vi "get_dequeue_buffer_element.vi"(8 "error in (no error)":errorcluster, 10 "continuous samples?":i32, 11 "SignalWriterMH110203USBStepperMotor in":refnum<class "SignalWriterMH110203USBStepperMotor.lvclass">) -> (0 "error out":errorcluster, 1 "finished?":bool, 2 "dequeued element":dbl, 3 "SignalWriterMH110203USBStepperMotor out":refnum<class "SignalWriterMH110203USBStepperMotor.lvclass">)   [LabVIEW 2010, in "SignalWriterMH110203USBStepperMotor.lvclass"]
uses:
  SignalWriterMH110203USBStepperMotor.lvclass
  SignalWriterMH110203USBStepperMotor.lvclass/SignalWriterMH110203USBStepperMotor.ctl
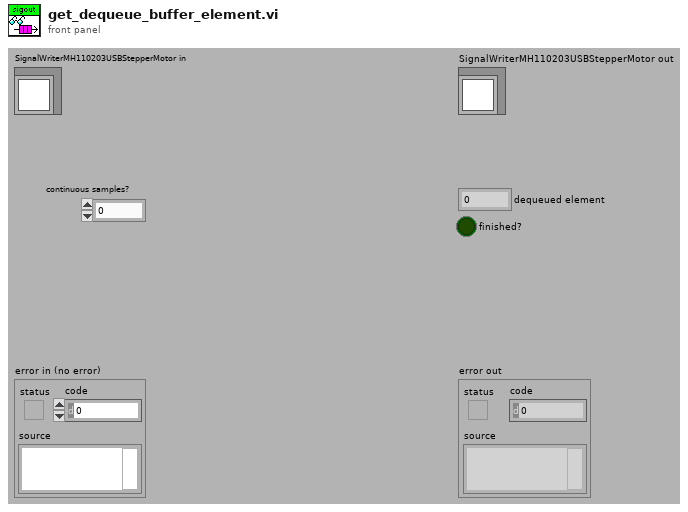
[diagram p1: front panel]
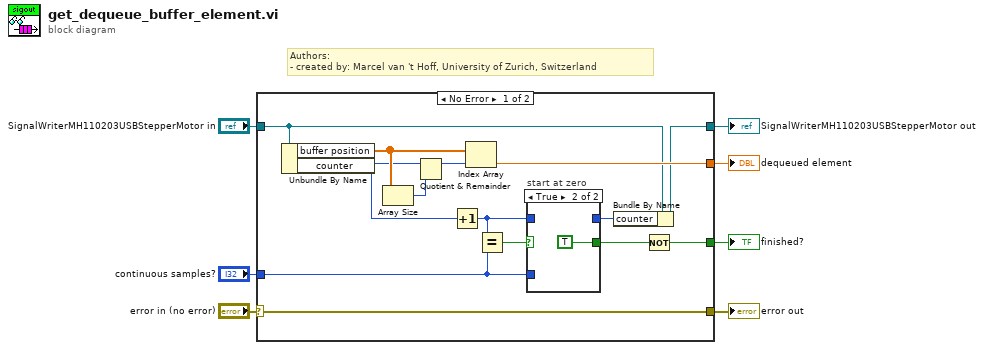
[diagram p0: block diagram]
diagram:
  # "Authors: \n- created by: Marcel van 't Hoff, University of Zurich, Switzerland"
  n1 = case shown="No Error" "error in (no error)" {
    selector: "error in (no error)" -> [w21 w25]
    tunnel: [w21 w25] -> w6
    tunnel: [w18 w24] -> w4
    tunnel: "SignalWriterMH110203USBStepperMotor in" -> [w19 w24]
    tunnel: [w20 _] -> w3
    tunnel: "continuous samples?" -> [w13 _]
    tunnel: [w14 _] -> w1
    frame No Error {
      n2 = Unbundle By Name(w19) -> ("buffer position"=w11:dbl[], "counter"=w9:i32)
      n3 = Array Size(array=w11) -> (size(s)=w10:i32)
      n4 = Quotient & Remainder(x=w9, y=w10) -> (x-y*floor(x/y)=w12:i32)  [unwired: 1 out]
      n5 = Increment(x=w9) -> (x+1=w8:i32)
      n6 = Index Array(array=w11, index=w12) -> (element=w20:dbl)
      n7 = Equal?(x=w8, y=w13) -> (x = y?=w17:bool)
      n8 = case "start at zero" shown="True" w17 {
        tunnel: w8 -> [w22 _]
        tunnel: [w22 _] -> w16
        tunnel: w13 -> [_ _]
        tunnel: [_ TRUE] -> w15
        frame False {
        }
        frame True {
        }
      }
      n9 = Bundle By Name(cluster=w19, "counter"=w16) -> (w18:refnum<class "SignalWriterMH110203USBStepperMotor.lvclass">)
      n10 = Not(x=w15) -> (.not. x?=w14:bool)
    }
    frame Error {
    }
  }
  "error out" <- w6
  "SignalWriterMH110203USBStepperMotor out" <- w4
  "dequeued element" <- w3
  "finished?" <- w1
